vi "LINX Digital Write Benchmark.vi"() -> ()   [LabVIEW 2013]
uses:
  <vilib>/LabVIEW Hacker/LINX/Private/Type Defs/Peripherals/Digital/Digital Write Control.ctl
  <vilib>/LabVIEW Hacker/LINX/Public/Peripherals/Digital/Digital Write 1 Chan.vi
  <vilib>/LabVIEW Hacker/LINX/LVH-LINX.lvlib
  <vilib>/ptbypt/NI_PtbyPt.lvlib
panel:
  in  "Stop Button 2":bool
  in  "Digital Values":T1[](array[typedef])=[{"Pin Number"=13, "Value"=TRUE}]
  out "Loop Rate":dbl(graph)
  out "Loop Time (ms)":i32
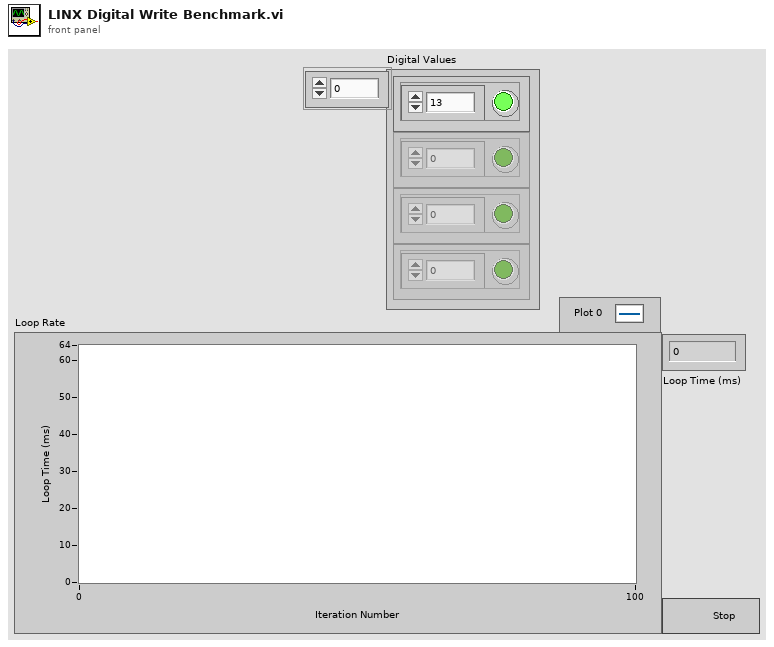
[diagram p1: front panel]
types:
  T1 = typedef "LVH-LINX.lvlib/Digital Write Control.ctl" = cluster{"Pin Number":u8, "Value":bool}
  T2 = typedef "LVH-LINX.lvlib/LINX Ref.ctl" = cluster{"Platform":T3, "Interface":T4, "LINX Device Config":T5}
  T3 = typedef "LVH-LINX.lvlib/Platform.ctl" = enum16{"LINX", "myRIO"}
  T4 = typedef "LVH-LINX.lvlib/Interface.ctl" = enum16{"Serial", "TCP"}
  T5 = typedef "LVH-LINX.lvlib/Device.lvlib/LINX Device Config.ctl" = cluster{"Interface":T4, "COM Port":refnum<visa-resource-name>, "TCP Configuration":T6, "Device Family":T7, "Device ID":u8, "Device Name":string, "TCP Ref":refnum<k5>}
  T6 = typedef "LVH-LINX.lvlib/Device.lvlib/TCP Config.ctl" = cluster{"IP Address":string, "Port":u16}
  T7 = typedef "LVH-LINX.lvlib/Device Family.ctl" = enum8{"National Instruments", "Digilent", "Arduino"}
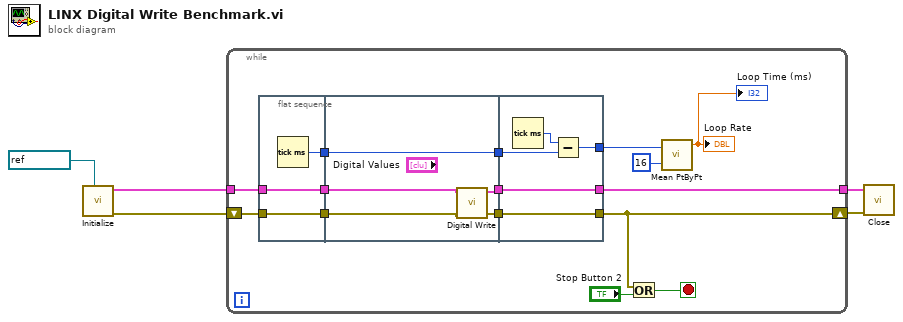
[diagram p0: block diagram]
diagram:
  n1 = call <vilib>:"Initialize.vi"("Serial Port"=refnum<visa-resource-name> "COM7") -> ("Error Out"=w4:errorcluster, "LINX Ref"=w3:T2)  [unwired: 8 in, 1 out]
  n2 = while {
    tunnel: w3 -> [w19]
    tunnel: [w18] -> w2
    shift-right: [w16] -> w1
    shift-left: w4 -> [w20]
    stop <- w17 stop-if-true
    n3 = flat-sequence {
      tunnel: w19 -> [w22]
      tunnel: w20 -> [w23]
      tunnel: [w23] -> w14
      tunnel: [w22] -> w13
      tunnel: [w21] -> w11
      tunnel: w14 -> [w24]
      tunnel: w13 -> [w27]
      tunnel: [w26] -> w12
      tunnel: w11 -> [w28]
      tunnel: [w28] -> w10
      tunnel: [w25] -> w6
      tunnel: [w32] -> w16
      tunnel: [w33] -> w18
      tunnel: w12 -> [w33]
      tunnel: w10 -> [w30]
      tunnel: [w29] -> w9
      tunnel: w6 -> [w32]
      frame #0 {
        n4 = Tick Count (ms)() -> (millisecond timer value=w21:u32)
      }
      frame #1 {
        n5 = call-poly <vilib>:"Digital Write.vi"("Error In"=w24, "LINX Resource"=w27) -> ("Error Out"=w25:errorcluster, "LINX Resource"=w26:T2)  [unwired: 8 in]
      }
      frame #2 {
        n6 = Tick Count (ms)() -> (millisecond timer value=w31:u32)
        n7 = Subtract(x=w31, y=w30) -> (x-y=w29:u32)
      }
    }
    n8 = Or(x=w16, y="Stop Button 2") -> (x .or. y?=w17:bool)
    n9 = call <vilib>:"Mean PtByPt.vi"("x"=w9, "sample length"=16) -> ("mean"=→"Loop Rate" →"Loop Time (ms)":dbl)  [unwired: 2 in, 1 out]
  }
  n10 = call <vilib>:"Close.vi"("Error In"=w1, "LINX Resource"=w2) -> ()  [unwired: 8 in, 2 out]
